vi "Stage.vi"() -> ()   [LabVIEW 2025]
uses:
  libximc.lvlib
panel:
  in  "Tab Control":T1(tab)=enum."Move Relative"
  in  "Controller 3":u16(ring) items=["xi-com:\\\\.\\COM4", "xi-com:\\\\.\\COM5", "xi-com:\\\\.\\COM6"]
  in  "Controller 2":u16(ring) items=["xi-com:\\\\.\\COM4", "xi-com:\\\\.\\COM5", "xi-com:\\\\.\\COM6"]
  in  "Controller 1":u16(ring) items=["xi-com:\\\\.\\COM4", "xi-com:\\\\.\\COM5", "xi-com:\\\\.\\COM6"]
  out "s/n 1":u32
  out "s/n 3":u32
  out "s/n 2":u32
  in  "Destination Y":i32
  in  "Destination Z":i32
  in  "Destination X":i32
  in  "Move To Destination":bool
  in  "Move Relative":bool
  in  "Shift Y":i32
  in  "Shift Z":i32
  in  "Shift X":i32
  in  "Shift Amount (Steps)":i32
  in  "shift stage":bool
  in  "Exit":bool
  out "Cursor X":dbl format="%#.2f"
  out "Cursor Z":dbl format="%#.2f"
  out "Cursor Y":dbl format="%#.2f"
  # "Position Status"
  # "Note: units of all positions are in steps."
  # "Initializes each motor in XILab."
  # "Controller IDs"
  # "Serial Numbers"
  # "Moves individual motors to desired height (units in steps)."
  # "Moves individual motors a number of steps."
  # "Moves all three motors the same amount of steps."
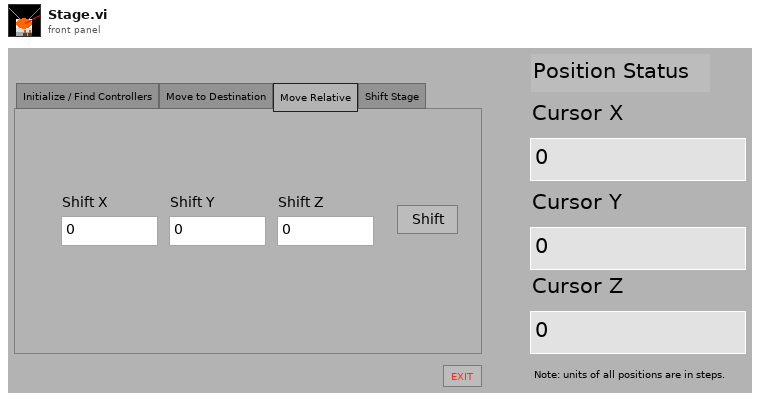
[diagram p1: front panel]
types:
  T1 = enum32{"Initialize / Find Controllers", "Move to Destination", "Move Relative", "Shift Stage"}
  T2 = enum32{"invalid app kind", "Development System", "Run Time System", "Student Edition", "Embedded LabVIEW", "Evaluation", "Custom"}
  T3 = cluster{"Number of controllers":i32, "Controllers' names":string[], "variant":variant, "quit":bool, "IDs":i32[]}
  T4 = cluster{"MoveSts":u32, "MvCmdSts":u32, "PWRSts":u32, "EncSts":u32, "WindSts":u32, "CurPosition":i32, "uCurPosition":i32, "@dummy control@":i8, "@dummy control@":i8, "@dummy control@":i8, "@dummy control@":i8, "EncPosition":i64, "CurSpeed":i32, "uCurSpeed":i32, "Ipwr":i32, "Upwr":i32, "Iusb":i32, "Uusb":i32, "CurT":i32, "Flags":u32, "GPIOFlags":u32, "CmdBufFreeSpace":u32}
  T5 = cluster{"Shift Y":i32, "Shift Z":i32, "Shift X":i32}
  T6 = cluster{"Destination Y":i32, "Destination Z":i32, "Destination X":i32}
  T7 = cluster{"Shift Amount (Steps)":i32, "Shift Amount (Steps)":i32, "Shift Amount (Steps)":i32}
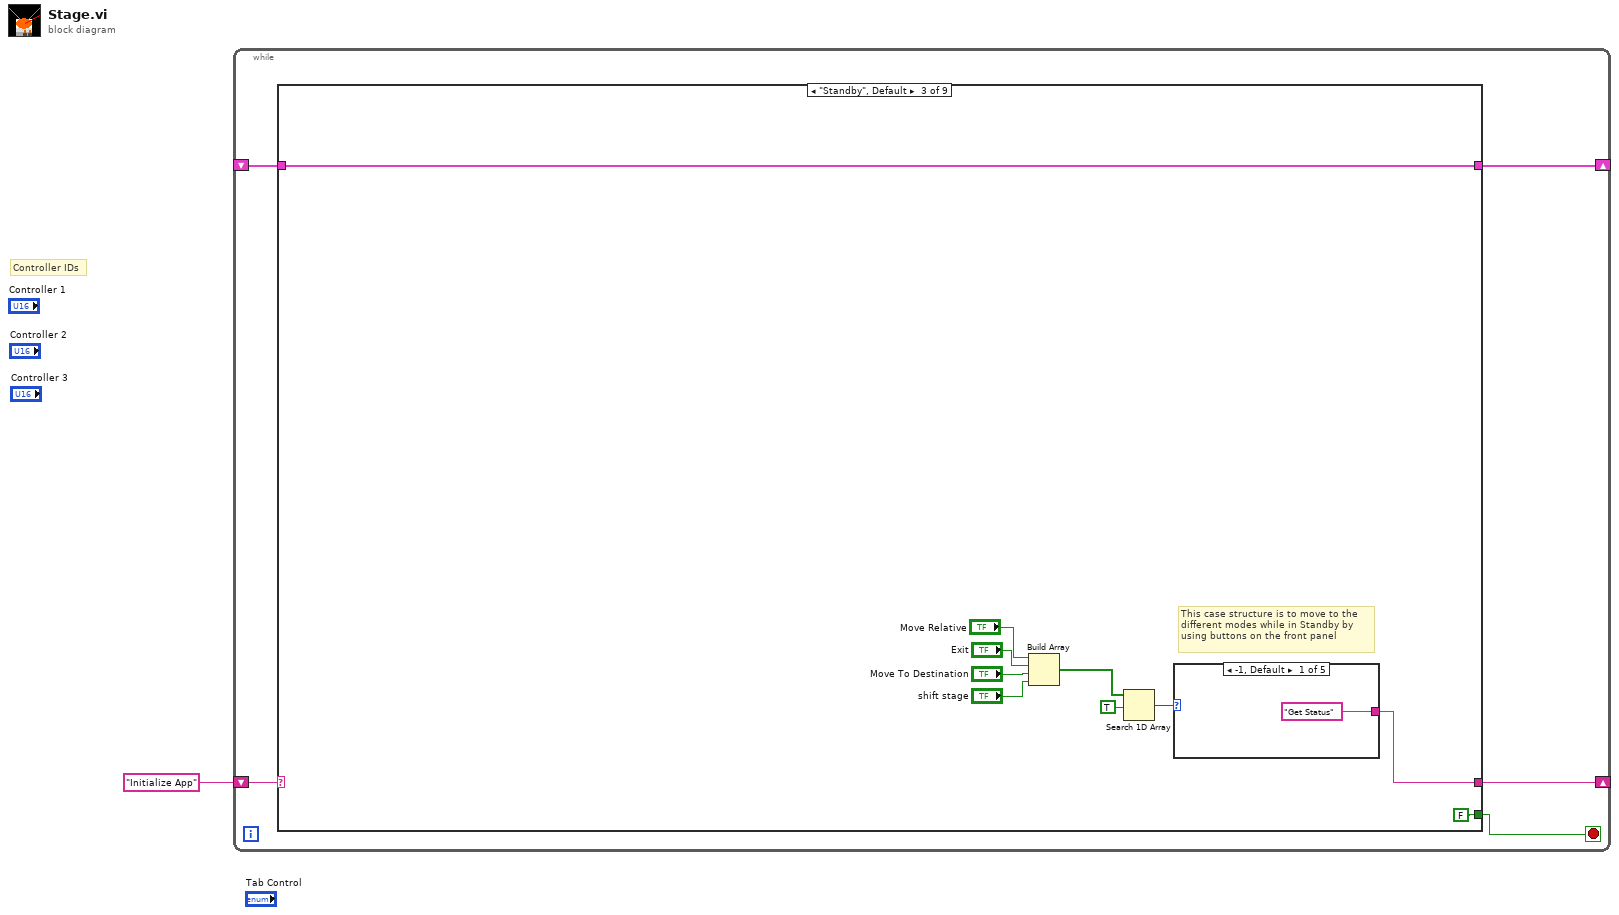
[diagram p0: block diagram]
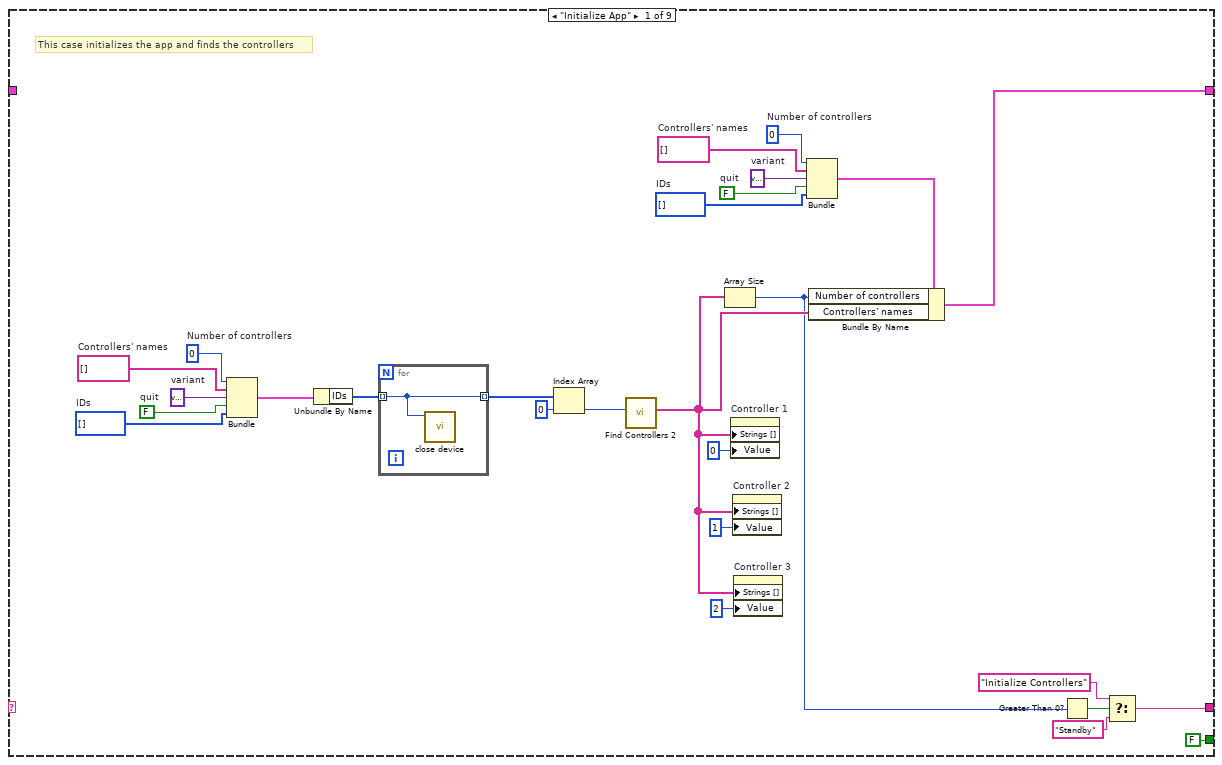
[diagram p2: hidden frame]
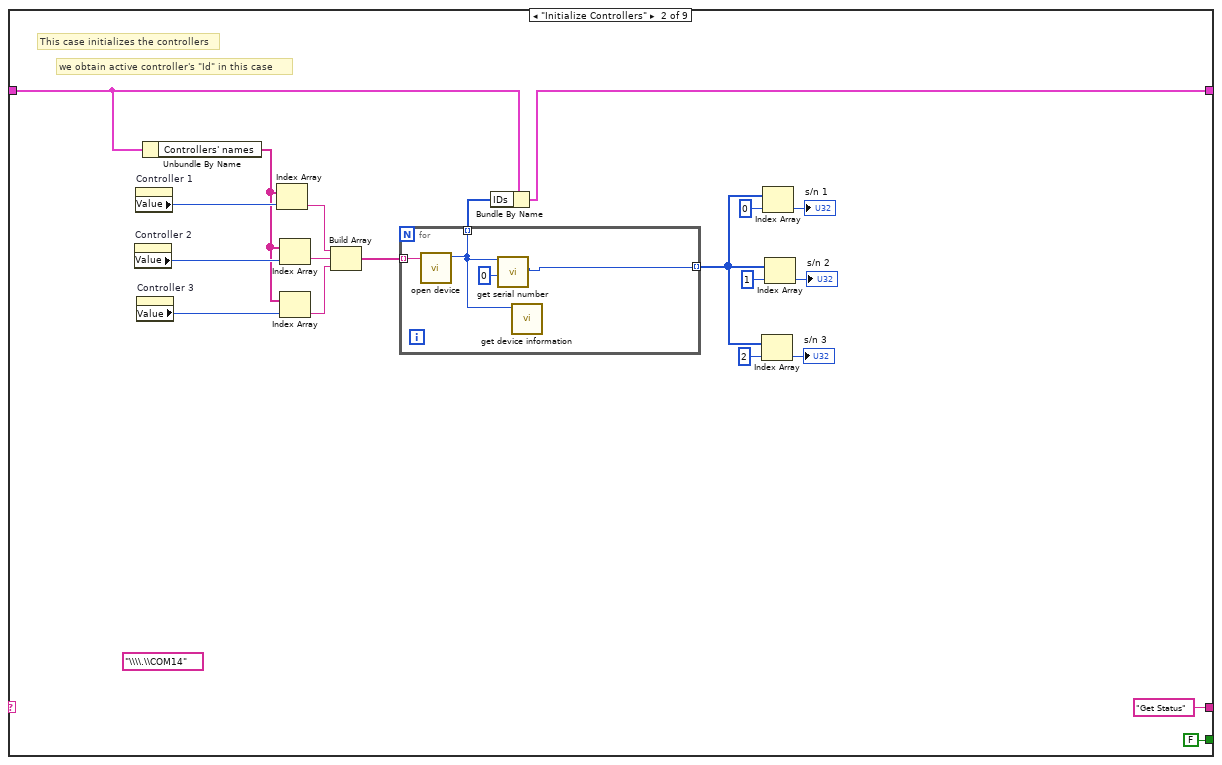
[diagram p3: hidden frame]
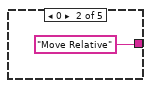
[diagram p4: hidden frame]
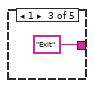
[diagram p5: hidden frame]
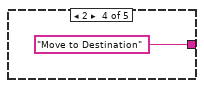
[diagram p6: hidden frame]
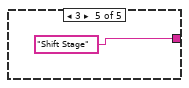
[diagram p7: hidden frame]
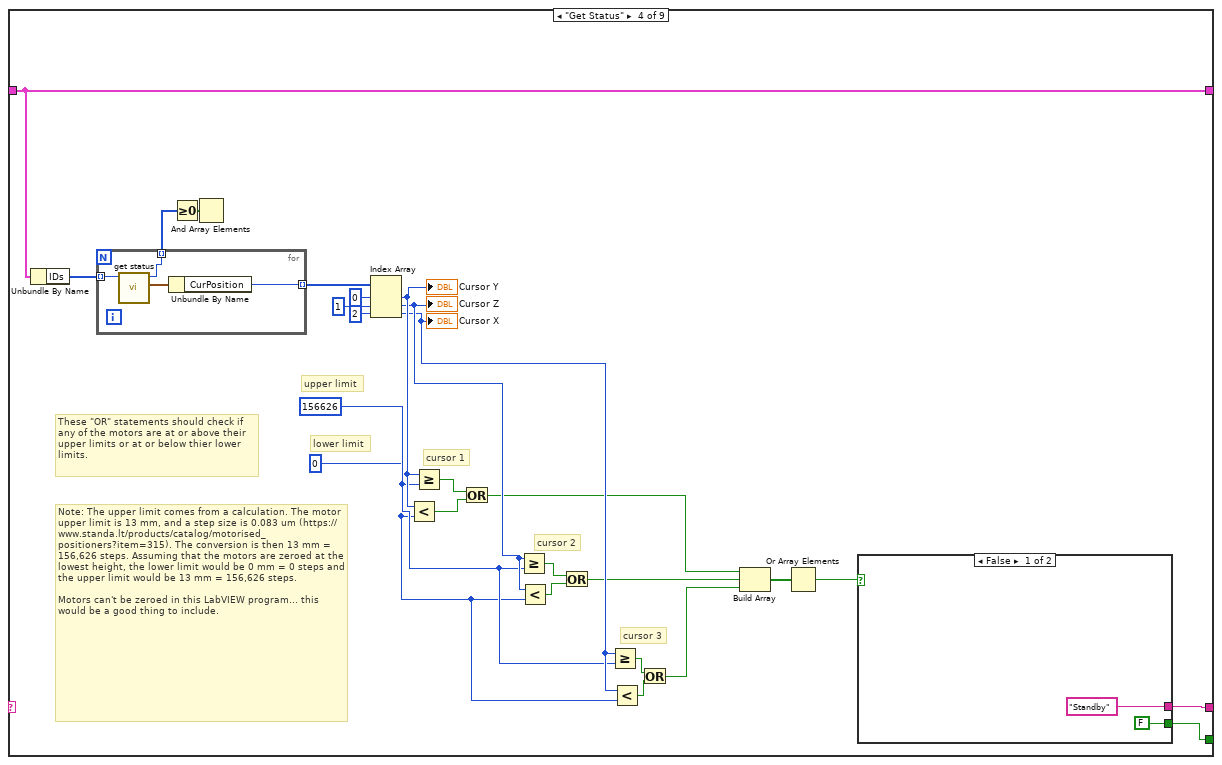
[diagram p8: hidden frame]
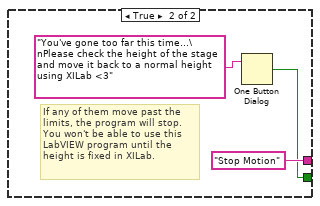
[diagram p9: hidden frame]
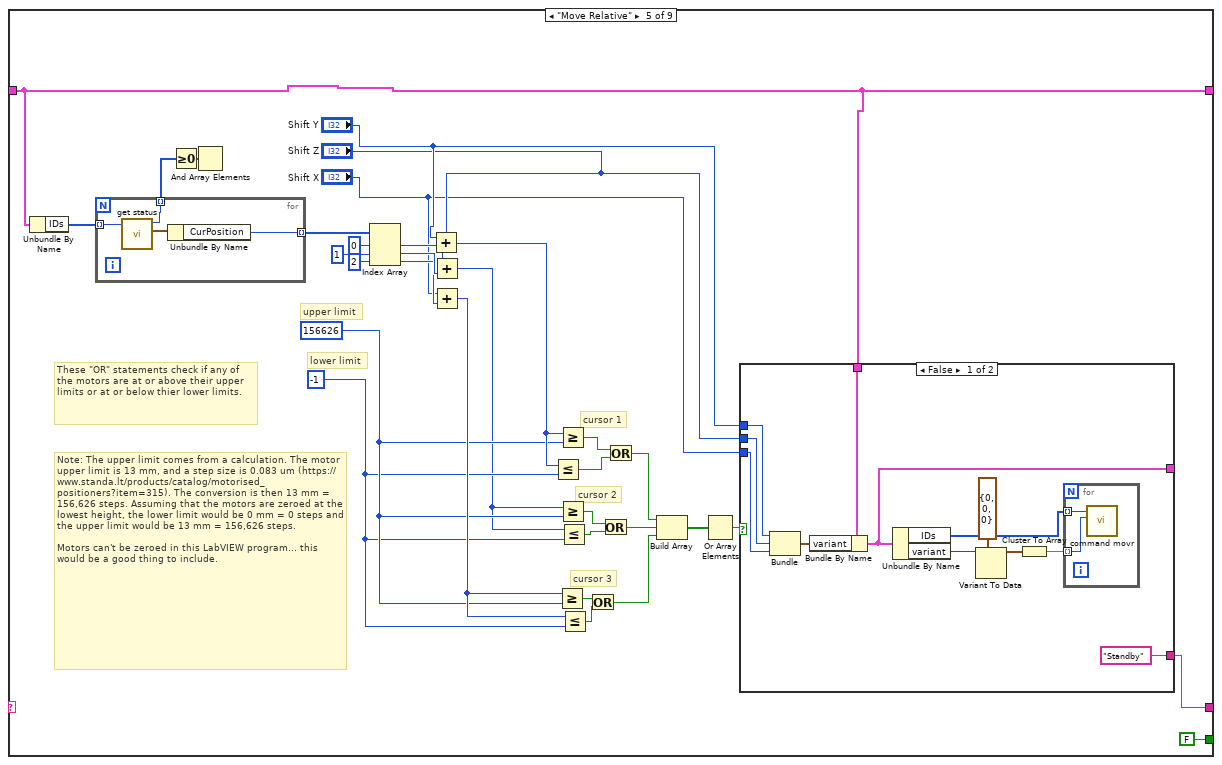
[diagram p10: hidden frame]
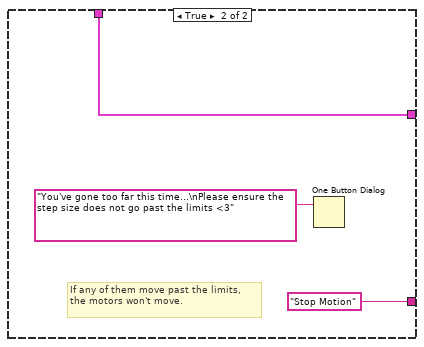
[diagram p11: hidden frame]
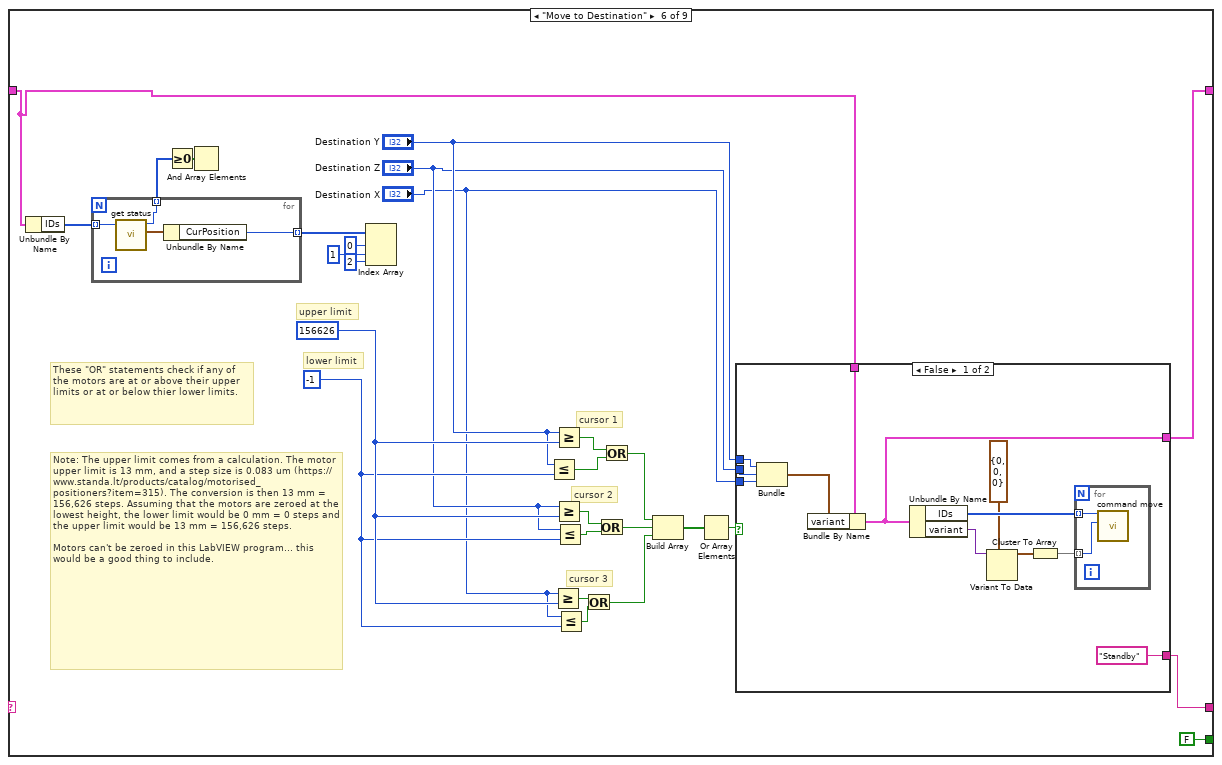
[diagram p12: hidden frame]
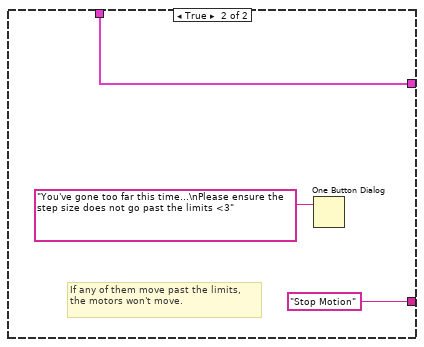
[diagram p13: hidden frame]
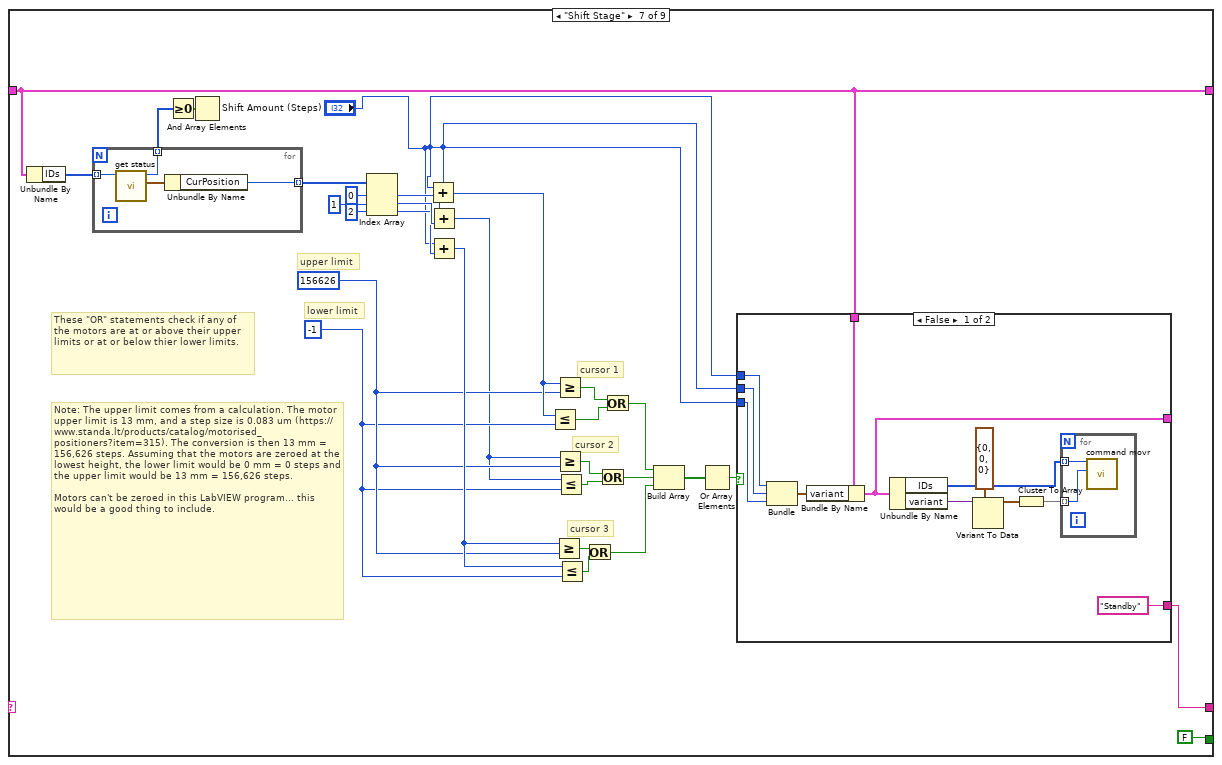
[diagram p14: hidden frame]
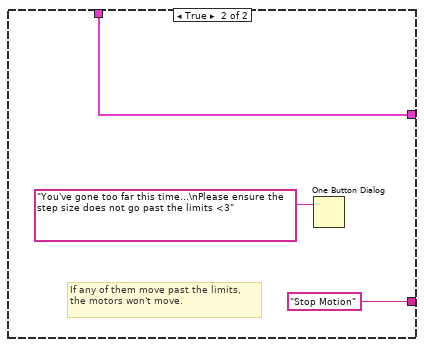
[diagram p15: hidden frame]
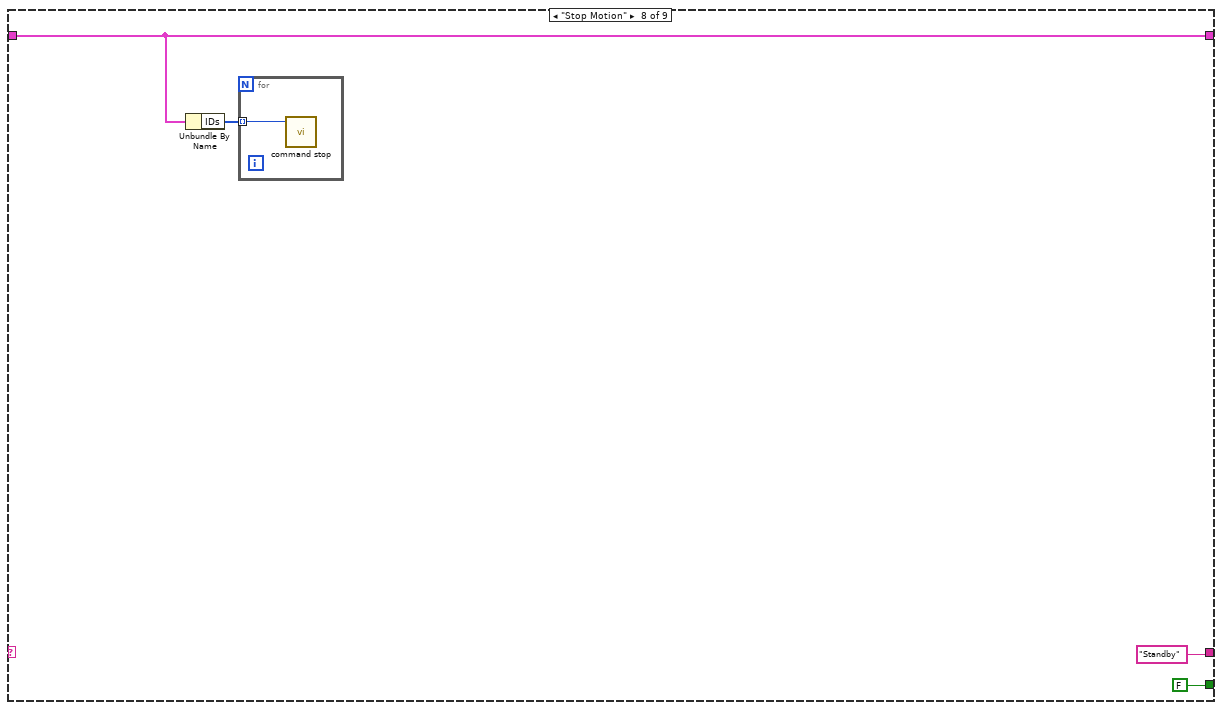
[diagram p16: hidden frame]
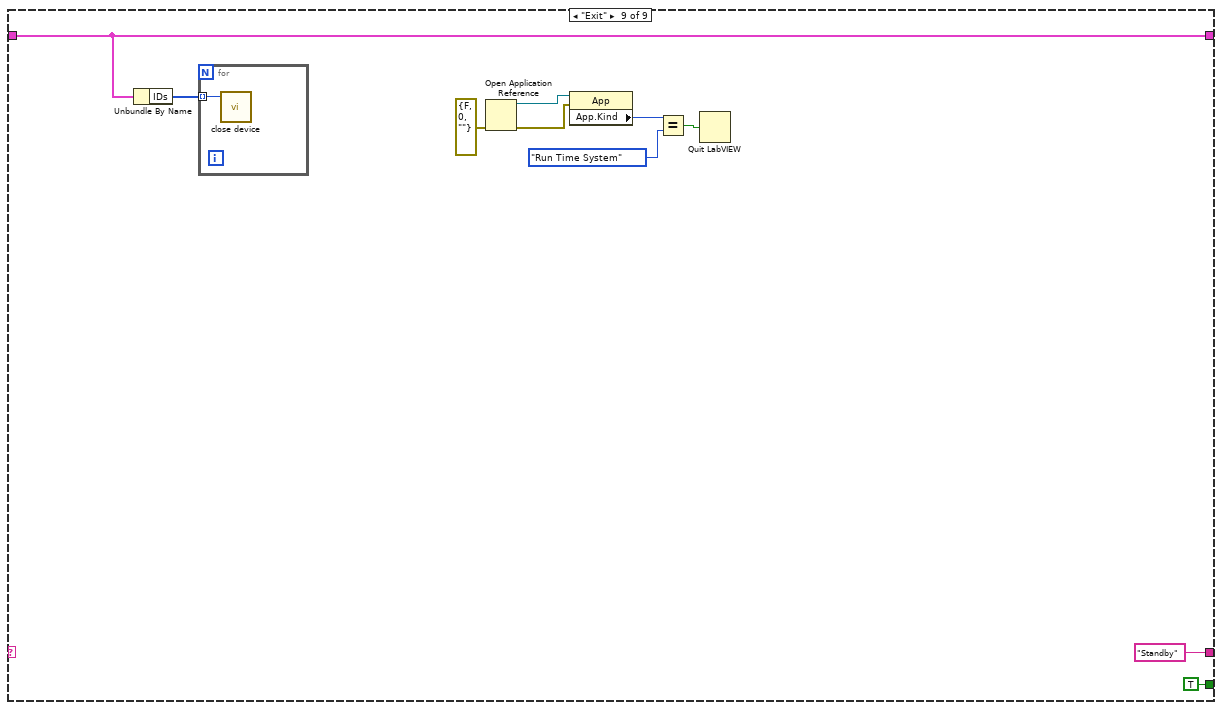
[diagram p17: hidden frame]
diagram:
  # "Controller IDs"
  n1 = while {
    shift-right: [w5] -> _
    shift-left: _ -> [w6]
    shift-right: [w4] -> _
    shift-left: "Initialize App" -> [w3]
    stop <- w2 stop-if-true
    n2 = case shown="\"Standby\", Default" w3 {
      tunnel: [w27 w44 w68 w92 w110 w167 w211 w261 w273] -> w5
      tunnel: w6 -> [_ w45 w68 w92 w110 w166 w211 w261 w273]
      tunnel: [w8 "Get Status" w62 w88 w109 w165 w210 "Standby" "Standby"] -> w4
      tunnel: [FALSE ("quit") FALSE ("quit") FALSE ("quit") w74 FALSE ("quit") FALSE ("quit") FALSE FALSE TRUE ("quit")] -> w2
      frame "Initialize App" {
        w14 = i32[] []  # IDs
        w15 = FALSE  # quit
        w16 = variant  # variant
        w17 = string[] []  # Controllers' names
        w18 = 0  # Number of controllers
        w29 = i32[] []  # IDs
        w30 = FALSE  # quit
        w31 = variant  # variant
        w32 = string[] []  # Controllers' names
        w33 = 0  # Number of controllers
        # "This case initializes the app and finds the controllers"
        n3 = Bundle("Number of controllers"=w18, "Controllers' names"=w17, "variant"=w16, "quit"=w15, "IDs"=w14) -> (w13:T3)  [unwired: 1 in]
        n4 = Unbundle By Name(w13) -> ("IDs"=w20:i32[])
        n5 = for {
          tunnel: w20 -> [w34] mode=indexing
          tunnel: [w34] -> w19 mode=indexing
          n6 = call "close device.vi"("id"=w34) -> ()  [unwired: 8 in, 3 out]
        }
        n7 = Index Array(array=w19, index=0) -> (element=w25:i32)
        n8 = call "Find Controllers 2.vi"("Numeric"=w25) -> ("Names"=w21:string[])  [unwired: 9 in, 1 out]
        n9 = Array Size(array=w21) -> (size(s)=w11:i32)
        n10 = property on="Controller 1" class="Ring (strict)"("Strings []"=w21, "Value"=0) -> ()  [unwired: 2 in, 2 out]
        n11 = property on="Controller 2" class="Ring (strict)"("Strings []"=w21, "Value"=1) -> ()  [unwired: 2 in, 2 out]
        n12 = property on="Controller 3" class="Ring (strict)"("Strings []"=w21, "Value"=2 ("Controller 3")) -> ()  [unwired: 2 in, 2 out]
        n13 = Bundle("Number of controllers"=w33, "Controllers' names"=w32, "variant"=w31, "quit"=w30, "IDs"=w29) -> (w28:T3)  [unwired: 1 in]
        n14 = Bundle By Name(cluster=w28, "Number of controllers"=w11, "Controllers' names"=w21) -> (w27:T3)
        n15 = Greater Than 0?(x=w11) -> (x > 0?=w12:bool)
        n16 = Select(t="Initialize Controllers", s=w12, f="Standby") -> (s? t:f=w8:string)
      }
      frame "Initialize Controllers" {
        (unwired) "\\\\.\\COM14" ("name")
        # "we obtain active controller's \"Id\" in this case"
        # "This case initializes the controllers"
        n17 = property on="Controller 2" class="Ring (strict)"() -> ("Value"=w53:u16)  [unwired: 2 in, 2 out]
        n18 = property on="Controller 1" class="Ring (strict)"() -> ("Value"=w54:u16)  [unwired: 2 in, 2 out]
        n19 = property on="Controller 3" class="Ring (strict)"() -> ("Value"=w52:u16)  [unwired: 2 in, 2 out]
        n20 = Unbundle By Name(w45) -> ("Controllers' names"=w48:string[])
        n21 = Index Array(array=w48, index=w54) -> (element=w49:string)
        n22 = Index Array(array=w48, index=w53) -> (element=w50:string)
        n23 = Index Array(array=w48, index=w52) -> (element=w51:string)
        n24 = Build Array(w49, w50, w51) -> (w47:string[])
        n25 = for {
          tunnel: w47 -> [w58] mode=indexing
          tunnel: [w56] -> w46 mode=indexing
          tunnel: [w55] -> w37 mode=indexing
          n26 = call "open device.vi"("uri"=w58) -> ("function return"=w56:i32)  [unwired: 9 in, 1 out]
          n27 = call "get serial number.vi"("SerialNumber"=0, "id"=w56) -> ("SerialNumber out"=w55:u32)  [unwired: 7 in, 2 out]
          n28 = call "get device information.vi"("id"=w56) -> ()  [unwired: 8 in, 3 out]
        }
        n29 = Bundle By Name(cluster=w45, "IDs"=w46) -> (w44:T3)
        n30 = Index Array(array=w37, index=u32 2 ("serial")) -> (element=→"s/n 3":u32)
        n31 = Index Array(array=w37, index=u32 0 ("serial")) -> (element=→"s/n 1":u32)
        n32 = Index Array(array=w37, index=u32 1 ("serial")) -> (element=→"s/n 2":u32)
      }
      frame "Standby", Default {
        # "This case structure is to move to the different modes while in Standby by using buttons on the front panel"
        n33 = Build Array("Move Relative", "Exit", "Move To Destination", "shift stage") -> (w65:bool[])
        n34 = Search 1D Array(1D array=w65, element=TRUE) -> (index of element=w63:i32)  [unwired: 1 in]
        n35 = case shown="-1, Default" w63 {
          tunnel: ["Get Status" "Move Relative" "Exit" "Move to Destination" "Shift Stage"] -> w62
          frame -1, Default {
          }
          frame 0 {
          }
          frame 1 {
          }
          frame 2 {
          }
          frame 3 {
          }
        }
      }
      frame "Get Status" {
        w75 = 0
        w76 = 156626
        # "cursor 3"
        # "cursor 2"
        # "cursor 1"
        # "lower limit"
        # "upper limit"
        # "Note: The upper limit comes from a calculation. The motor upper limit is 13 mm, and a step size is 0.083 um (https://www.standa.lt/products/catalog/motorised_positioners?item=315). The conversion is then 13 mm = 156,626 steps. Assuming that the motors are zeroed at the lowest height, the lower limit would be 0 mm = 0 steps and the upper limit would be 13 mm = 156,626 steps.\n\nMotors can't be zeroed in this LabVIEW program... this would be a good thing to include."
        # "These \"OR\" statements should check if any of the motors are at or above their upper limits or at or below thier lower limits."
        n36 = Unbundle By Name(w92) -> ("IDs"=w99:i32[])
        n37 = for {
          tunnel: [w108] -> w97 mode=indexing
          tunnel: w99 -> [w107] mode=indexing
          tunnel: [w106] -> w98 mode=indexing
          n38 = call "get status.vi"("id"=w107) -> ("status out"=w105:T4, "function return"=w106:i32)  [unwired: 8 in, 1 out]
          n39 = Unbundle By Name(w105) -> ("CurPosition"=w108:i32)
        }
        n40 = Greater Or Equal To 0?(x=w98) -> (x >= 0?=w93:bool[])
        n41 = And Array Elements(Boolean array=w93) -> ()  [unwired: 1 out]
        n42 = Index Array(array=w97, index #1=0 ("index"), index #2=1 ("index"), index #3=2 ("index")) -> (element #1=w90:i32, element #2=w83:i32, element #3=w82:i32)
        "Cursor Y" <- w90
        "Cursor Z" <- w83
        "Cursor X" <- w82
        n43 = Less?(x=w90, y=w75) -> (x < y?=w89:bool)
        n44 = Greater Or Equal?(x=w90, y=w76) -> (x >= y?=w91:bool)
        n45 = Or(x=w91, y=w89) -> (x .or. y?=w81:bool)
        n46 = Greater Or Equal?(x=w83, y=w76) -> (x >= y?=w87:bool)
        n47 = Less?(x=w83, y=w75) -> (x < y?=w86:bool)
        n48 = Or(x=w87, y=w86) -> (x .or. y?=w80:bool)
        n49 = Greater Or Equal?(x=w82, y=w76) -> (x >= y?=w85:bool)
        n50 = Less?(x=w82, y=w75) -> (x < y?=w84:bool)
        n51 = Or(x=w85, y=w84) -> (x .or. y?=w79:bool)
        n52 = Build Array(w81, w80, w79) -> (w78:bool[])
        n53 = Or Array Elements(Boolean array=w78) -> (logical OR=w77:bool)
        n54 = case shown="False" w77 {
          tunnel: ["Standby" "Stop Motion"] -> w88
          tunnel: [FALSE w102] -> w74
          frame False {
          }
          frame True {
            # "If any of them move past the limits, the program will stop. You won't be able to use this LabVIEW program until the height is fixed in XILab."
            n55 = One Button Dialog(message="You've gone too far this time...\nPlease check the height of the stage and move it back to a normal height using XILab <3") -> (true=w102:bool)  [unwired: 1 in]
          }
        }
      }
      frame "Move Relative" {
        w115 = -1
        w116 = 156626
        # "cursor 3"
        # "cursor 2"
        # "cursor 1"
        # "lower limit"
        # "upper limit"
        # "Note: The upper limit comes from a calculation. The motor upper limit is 13 mm, and a step size is 0.083 um (https://www.standa.lt/products/catalog/motorised_positioners?item=315). The conversion is then 13 mm = 156,626 steps. Assuming that the motors are zeroed at the lowest height, the lower limit would be 0 mm = 0 steps and the upper limit would be 13 mm = 156,626 steps.\n\nMotors can't be zeroed in this LabVIEW program... this would be a good thing to include."
        # "These \"OR\" statements check if any of the motors are at or above their upper limits or at or below thier lower limits."
        n56 = Unbundle By Name(w110) -> ("IDs"=w139:i32[])
        n57 = for {
          tunnel: [w161] -> w137 mode=indexing
          tunnel: w139 -> [w160] mode=indexing
          tunnel: [w159] -> w138 mode=indexing
          n58 = call "get status.vi"("id"=w160) -> ("status out"=w158:T4, "function return"=w159:i32)  [unwired: 8 in, 1 out]
          n59 = Unbundle By Name(w158) -> ("CurPosition"=w161:i32)
        }
        n60 = Greater Or Equal To 0?(x=w138) -> (x >= 0?=w133:bool[])
        n61 = And Array Elements(Boolean array=w133) -> ()  [unwired: 1 out]
        n62 = Index Array(array=w137, index #1=0 ("index"), index #2=1 ("index"), index #3=2 ("index")) -> (element #1=w121:i32, element #2=w120:i32, element #3=w119:i32)
        n63 = Add(x="Shift Y", y=w121) -> (x+y=w118:i32)
        n64 = Add(x="Shift Z", y=w120) -> (x+y=w114:i32)
        n65 = Add(x="Shift X", y=w119) -> (x+y=w117:i32)
        n66 = Less Or Equal?(x=w118, y=w115) -> (x <= y?=w131:bool)
        n67 = Greater Or Equal?(x=w117, y=w116) -> (x >= y?=w128:bool)
        n68 = Greater Or Equal?(x=w118, y=w116) -> (x >= y?=w132:bool)
        n69 = Greater Or Equal?(x=w114, y=w116) -> (x >= y?=w130:bool)
        n70 = Less Or Equal?(x=w114, y=w115) -> (x <= y?=w129:bool)
        n71 = Less Or Equal?(x=w117, y=w115) -> (x <= y?=w127:bool)
        n72 = Or(x=w128, y=w127) -> (x .or. y?=w124:bool)
        n73 = Or(x=w130, y=w129) -> (x .or. y?=w125:bool)
        n74 = Or(x=w132, y=w131) -> (x .or. y?=w126:bool)
        n75 = Build Array(w126, w125, w124) -> (w123:bool[])
        n76 = Or Array Elements(Boolean array=w123) -> (logical OR=w122:bool)
        n77 = case shown="False" w122 {
          tunnel: ["Standby" "Stop Motion"] -> w109
          tunnel: "Shift Y" -> [w151 _]
          tunnel: "Shift Z" -> [w150 _]
          tunnel: "Shift X" -> [w149 _]
          tunnel: w110 -> [w148 w155]
          tunnel: [w146 w155] -> _
          frame False {
            n78 = Bundle("Shift Y"=w151, "Shift Z"=w150, "Shift X"=w149) -> (w147:T5)  [unwired: 1 in]
            n79 = Bundle By Name(cluster=w148, "variant"=w147) -> (w146:T3)
            n80 = Unbundle By Name(w146) -> ("IDs"=w141:i32[], "variant"=w143:variant)
            n81 = Variant To Data(type=cluster{u32, u32, u32} {0, 0, 0}, Variant=w143) -> (data=w144:cluster{u32, u32, u32})  [unwired: 1 in, 1 out]
            n82 = Cluster To Array(cluster=w144) -> (array=w145:u32[])
            n83 = for {
              tunnel: w145 -> [w153] mode=indexing
              tunnel: w141 -> [w154] mode=indexing
              n84 = call "command movr.vi"("DeltaPosition"=w153, "id"=w154) -> ()  [unwired: 8 in, 2 out]
            }
          }
          frame True {
            # "If any of them move past the limits, the motors won't move."
            n85 = One Button Dialog(message="You've gone too far this time...\nPlease ensure the step size does not go past the limits <3") -> ()  [unwired: 1 in, 1 out]
          }
        }
      }
      frame "Move to Destination" {
        w168 = -1
        w169 = 156626
        # "cursor 3"
        # "cursor 2"
        # "cursor 1"
        # "lower limit"
        # "upper limit"
        # "Note: The upper limit comes from a calculation. The motor upper limit is 13 mm, and a step size is 0.083 um (https://www.standa.lt/products/catalog/motorised_positioners?item=315). The conversion is then 13 mm = 156,626 steps. Assuming that the motors are zeroed at the lowest height, the lower limit would be 0 mm = 0 steps and the upper limit would be 13 mm = 156,626 steps.\n\nMotors can't be zeroed in this LabVIEW program... this would be a good thing to include."
        # "These \"OR\" statements check if any of the motors are at or above their upper limits or at or below thier lower limits."
        n86 = Unbundle By Name(w166) -> ("IDs"=w187:i32[])
        n87 = for {
          tunnel: [w209] -> w185 mode=indexing
          tunnel: w187 -> [w208] mode=indexing
          tunnel: [w207] -> w186 mode=indexing
          n88 = call "get status.vi"("id"=w208) -> ("status out"=w206:T4, "function return"=w207:i32)  [unwired: 8 in, 1 out]
          n89 = Unbundle By Name(w206) -> ("CurPosition"=w209:i32)
        }
        n90 = Greater Or Equal To 0?(x=w186) -> (x >= 0?=w181:bool[])
        n91 = And Array Elements(Boolean array=w181) -> ()  [unwired: 1 out]
        n92 = Index Array(array=w185, index #1=0 ("index"), index #2=1 ("index"), index #3=2 ("index")) -> ()  [unwired: 3 out]
        n93 = Less Or Equal?(x="Destination Y", y=w168) -> (x <= y?=w179:bool)
        n94 = Greater Or Equal?(x="Destination X", y=w169) -> (x >= y?=w176:bool)
        n95 = Greater Or Equal?(x="Destination Y", y=w169) -> (x >= y?=w180:bool)
        n96 = Greater Or Equal?(x="Destination Z", y=w169) -> (x >= y?=w178:bool)
        n97 = Less Or Equal?(x="Destination Z", y=w168) -> (x <= y?=w177:bool)
        n98 = Less Or Equal?(x="Destination X", y=w168) -> (x <= y?=w175:bool)
        n99 = Or(x=w176, y=w175) -> (x .or. y?=w172:bool)
        n100 = Or(x=w178, y=w177) -> (x .or. y?=w173:bool)
        n101 = Or(x=w180, y=w179) -> (x .or. y?=w174:bool)
        n102 = Build Array(w174, w173, w172) -> (w171:bool[])
        n103 = Or Array Elements(Boolean array=w171) -> (logical OR=w170:bool)
        n104 = case shown="False" w170 {
          tunnel: ["Standby" "Stop Motion"] -> w165
          tunnel: "Destination Y" -> [w193 _]
          tunnel: "Destination Z" -> [w192 _]
          tunnel: "Destination X" -> [w191 _]
          tunnel: w166 -> [w190 w203]
          tunnel: [w189 w203] -> w167
          frame False {
            n105 = Bundle("Destination Y"=w193, "Destination Z"=w192, "Destination X"=w191) -> (w195:T6)  [unwired: 1 in]
            n106 = Bundle By Name(cluster=w190, "variant"=w195) -> (w189:T3)
            n107 = Unbundle By Name(w189) -> ("IDs"=w197:i32[], "variant"=w199:variant)
            n108 = Variant To Data(type=cluster{u32, u32, u32} {0, 0, 0}, Variant=w199) -> (data=w196:cluster{u32, u32, u32})  [unwired: 1 in, 1 out]
            n109 = Cluster To Array(cluster=w196) -> (array=w198:u32[])
            n110 = for {
              tunnel: w198 -> [w201] mode=indexing
              tunnel: w197 -> [w202] mode=indexing
              n111 = call "command move.vi"("Position"=w201, "id"=w202) -> ()  [unwired: 8 in, 2 out]
            }
          }
          frame True {
            # "If any of them move past the limits, the motors won't move."
            n112 = One Button Dialog(message="You've gone too far this time...\nPlease ensure the step size does not go past the limits <3") -> ()  [unwired: 1 in, 1 out]
          }
        }
      }
      frame "Shift Stage" {
        w214 = -1
        w215 = 156626
        # "cursor 3"
        # "cursor 2"
        # "cursor 1"
        # "lower limit"
        # "upper limit"
        # "Note: The upper limit comes from a calculation. The motor upper limit is 13 mm, and a step size is 0.083 um (https://www.standa.lt/products/catalog/motorised_positioners?item=315). The conversion is then 13 mm = 156,626 steps. Assuming that the motors are zeroed at the lowest height, the lower limit would be 0 mm = 0 steps and the upper limit would be 13 mm = 156,626 steps.\n\nMotors can't be zeroed in this LabVIEW program... this would be a good thing to include."
        # "These \"OR\" statements check if any of the motors are at or above their upper limits or at or below thier lower limits."
        n113 = Unbundle By Name(w211) -> ("IDs"=w238:i32[])
        n114 = for {
          tunnel: [w260] -> w236 mode=indexing
          tunnel: w238 -> [w259] mode=indexing
          tunnel: [w258] -> w237 mode=indexing
          n115 = call "get status.vi"("id"=w259) -> ("status out"=w257:T4, "function return"=w258:i32)  [unwired: 8 in, 1 out]
          n116 = Unbundle By Name(w257) -> ("CurPosition"=w260:i32)
        }
        n117 = Greater Or Equal To 0?(x=w237) -> (x >= 0?=w232:bool[])
        n118 = And Array Elements(Boolean array=w232) -> ()  [unwired: 1 out]
        n119 = Index Array(array=w236, index #1=0 ("index"), index #2=1 ("index"), index #3=2 ("index")) -> (element #1=w220:i32, element #2=w219:i32, element #3=w218:i32)
        n120 = Add(x="Shift Amount (Steps)", y=w220) -> (x+y=w217:i32)
        n121 = Add(x="Shift Amount (Steps)", y=w219) -> (x+y=w213:i32)
        n122 = Add(x="Shift Amount (Steps)", y=w218) -> (x+y=w216:i32)
        n123 = Less Or Equal?(x=w217, y=w214) -> (x <= y?=w230:bool)
        n124 = Greater Or Equal?(x=w216, y=w215) -> (x >= y?=w227:bool)
        n125 = Greater Or Equal?(x=w217, y=w215) -> (x >= y?=w231:bool)
        n126 = Greater Or Equal?(x=w213, y=w215) -> (x >= y?=w229:bool)
        n127 = Less Or Equal?(x=w213, y=w214) -> (x <= y?=w228:bool)
        n128 = Less Or Equal?(x=w216, y=w214) -> (x <= y?=w226:bool)
        n129 = Or(x=w227, y=w226) -> (x .or. y?=w223:bool)
        n130 = Or(x=w229, y=w228) -> (x .or. y?=w224:bool)
        n131 = Or(x=w231, y=w230) -> (x .or. y?=w225:bool)
        n132 = Build Array(w225, w224, w223) -> (w222:bool[])
        n133 = Or Array Elements(Boolean array=w222) -> (logical OR=w221:bool)
        n134 = case shown="False" w221 {
          tunnel: ["Standby" "Stop Motion"] -> w210
          tunnel: "Shift Amount (Steps)" -> [w250 _]
          tunnel: "Shift Amount (Steps)" -> [w249 _]
          tunnel: "Shift Amount (Steps)" -> [w248 _]
          tunnel: w211 -> [w247 w254]
          tunnel: [w245 w254] -> _
          frame False {
            n135 = Bundle("Shift Amount (Steps)"=w250, "Shift Amount (Steps)"=w249, "Shift Amount (Steps)"=w248) -> (w246:T7)  [unwired: 1 in]
            n136 = Bundle By Name(cluster=w247, "variant"=w246) -> (w245:T3)
            n137 = Unbundle By Name(w245) -> ("IDs"=w240:i32[], "variant"=w242:variant)
            n138 = Variant To Data(type=cluster{u32, u32, u32} {0, 0, 0}, Variant=w242) -> (data=w243:cluster{u32, u32, u32})  [unwired: 1 in, 1 out]
            n139 = Cluster To Array(cluster=w243) -> (array=w244:u32[])
            n140 = for {
              tunnel: w244 -> [w252] mode=indexing
              tunnel: w240 -> [w253] mode=indexing
              n141 = call "command movr.vi"("DeltaPosition"=w252, "id"=w253) -> ()  [unwired: 8 in, 2 out]
            }
          }
          frame True {
            # "If any of them move past the limits, the motors won't move."
            n142 = One Button Dialog(message="You've gone too far this time...\nPlease ensure the step size does not go past the limits <3") -> ()  [unwired: 1 in, 1 out]
          }
        }
      }
      frame "Stop Motion" {
        n143 = Unbundle By Name(w261) -> ("IDs"=w262:i32[])
        n144 = for {
          tunnel: w262 -> [w265] mode=indexing
          n145 = call "command stop.vi"("id"=w265) -> ()  [unwired: 9 in, 2 out]
        }
      }
      frame "Exit" {
        n146 = Unbundle By Name(w273) -> ("IDs"=w275:i32[])
        n147 = for {
          tunnel: w275 -> [w276] mode=indexing
          n148 = call "close device.vi"("id"=w276) -> ()  [unwired: 8 in, 3 out]
        }
        n149 = Open Application Reference(8:errorcluster {"status"=FALSE, "code"=0, "source"=""} ("error in (no error)")) -> (0:w266:errorcluster, 3:w267:refnum<vi>)  [unwired: 3 in]
        n150 = property class="App"(reference=w267, error in=w266) -> ("App.Kind"=w270:T2)  [unwired: 2 out]
        n151 = Equal?(x=w270, y=T2."Run Time System" ("Application:Kind")) -> (x = y?=w268:bool)
        n152 = Quit LabVIEW(quit? (T)=w268) -> ()
      }
    }
  }
